vi "GetSensorNodesFromAsset.vi"(8 "error in (no error)":errorcluster, 10 "Asset ID":string, 11 "ICM Service in":refnum<class "IcmMessageService.lvclass">) -> (0 "error out":errorcluster, 3 "SensorNodes":T1[](array[typedef]))   [LabVIEW 2017]
uses:
  <vilib>/addons/InsightCM/MessageBus/MessageService/IcmMessageService.lvclass
  <vilib>/addons/InsightCM/MessageBus/Base/controls/AssetNodeView.ctl
  <vilib>/addons/InsightCM/MessageBus/Base/controls/AssetState.ctl
  <vilib>/addons/InsightCM/MessageBus/Base/controls/Metric.ctl
  <vilib>/addons/InsightCM/MessageBus/Base/controls/KeyValuePair.ctl
  <vilib>/addons/InsightCM/MessageBus/Base/controls/AssetNodeReference.ctl
  <vilib>/addons/InsightCM/Utilities/DeviceModelHelpers/DeviceModelHelpers.lvlib
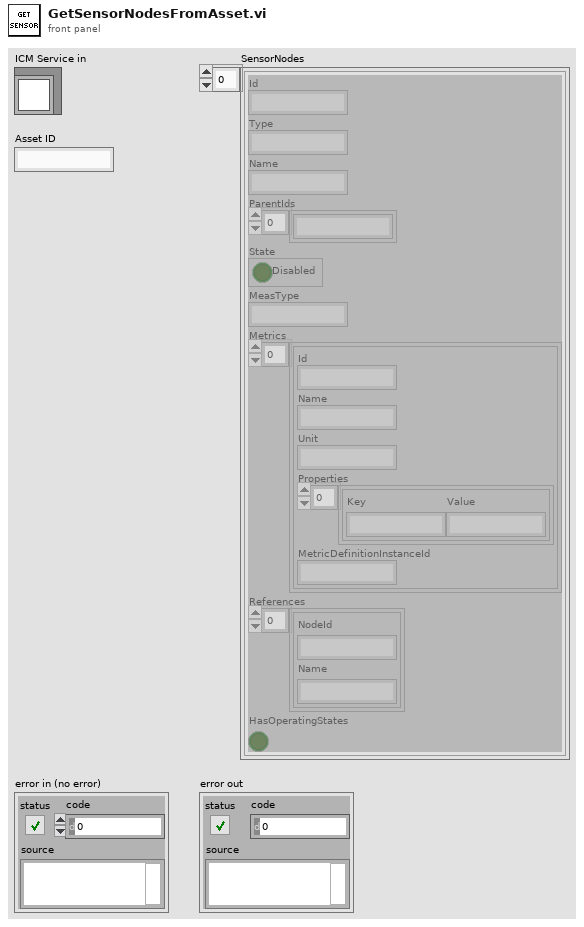
[diagram p1: front panel]
types:
  T1 = typedef "AssetNodeView.ctl" = cluster{"Id":string, "Type":string, "Name":string, "ParentIds":string[], "State":T2, "MeasType":string, "Metrics":T3[], "References":T5[], "HasOperatingStates":bool}
  T2 = typedef "AssetState.ctl" = cluster{"Disabled":bool}
  T3 = typedef "Metric.ctl" = cluster{"Id":string, "Name":string, "Unit":string, "Properties":T4[], "MetricDefinitionInstanceId":string}
  T4 = typedef "KeyValuePair.ctl" = cluster{"Key":string, "Value":string}
  T5 = typedef "AssetNodeReference.ctl" = cluster{"NodeId":string, "Name":string}
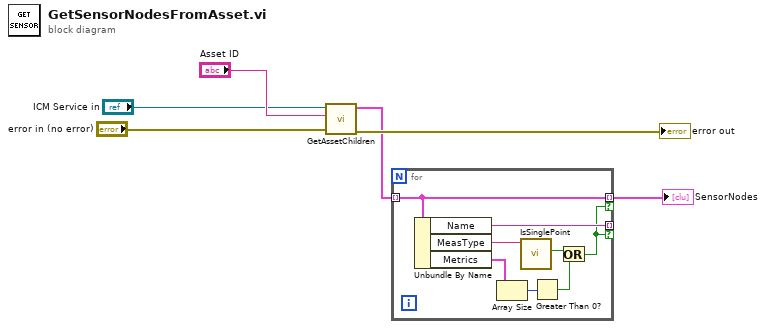
[diagram p0: block diagram]
diagram:
  n1 = call "GetAssetChildren.vi"("error in (no error)"="error in (no error)", "parent id"="Asset ID", "service"="ICM Service in") -> ("error out"=→"error out":errorcluster, "AssetNodes"=w1:T1[])  [unwired: 7 in]
  n2 = for {
    tunnel: w1 -> [w13] mode=indexing
    tunnel: [w13] -> w2 mode=indexing if=w7
    tunnel: [w8] -> _ mode=indexing if=w7
    n3 = Unbundle By Name(w13) -> ("Name"=w8:string, "MeasType"=w14:string, "Metrics"=w9:T3[])
    n4 = Array Size(array=w9) -> (size(s)=w11:i32)
    n5 = call <vilib>:"IsSinglePoint.vi"("MeasType"=w14) -> ("is single point"=w12:bool)  [unwired: 10 in]
    n6 = Greater Than 0?(x=w11) -> (x > 0?=w10:bool)
    n7 = Or(x=w12, y=w10) -> (x .or. y?=w7:bool)
  }
  "SensorNodes" <- w2
